vi "ni579x Synchronization Registers.vi"(0 "register instruction":T3, 5 "sync.resources":T1) -> (4 "read completion":T2, 14 "ready for input":bool)   [LabVIEW 2015, in "ni579x Synchronization v2 FPGA.lvlib"]
doc: "Set/get the configuration values for the Synchronization library by connecting it to the Register Bus.\n\n<B>Input Parameters</B>\n\n<B>register instruction</B> specifies a read or write register instruction. This parameter is usually obtained from the 'register instruction' parameter of the Process VI in the Register Bus FPGA library. The source of this parameter defines the instances of the Register Bus library to which the Synchronization library instance is wired, and is communicated from the host.\n\n<B>sync.resources</B> identifies the Synchronization instance. 'sync.resources' is obtained from the ni579x Create VI of this library.\n\n<B>Output Parameters</B>\n\n<B>read completion</B> indicates whether the register read operation has completed and returns the value for the register read.\n\n<B>ready for input</B> indicates whether the VI is ready to accept new input data in the next cycle. Use a Feedback Node to wire this parameter to the 'ready for output' terminal of an upstream node."
uses:
  <instrlib>/ni579x/Synchronization/v2/FPGA/ni579x Synchronization v2 FPGA.lvlib
  <instrlib>/_niInstr/Register Bus/v1/FPGA/Public/Register Instruction.ctl
  <instrlib>/_niInstr/Register Bus/v1/FPGA/Public/Read Completion.ctl
  <instrlib>/ni579x/Synchronization/v2/FPGA/Implementation/Resources.ctl
  <instrlib>/ni579x/Config/v2/Shared/Types/ni579x Register Bus Subsystem ID.ctl
  <instrlib>/_niInstr/Register Bus/v1/FPGA/niInstr Register Bus v1 FPGA.lvlib
  <instrlib>/ni579x/Config/v2/Shared/ni579x Config v2 Shared.lvlib
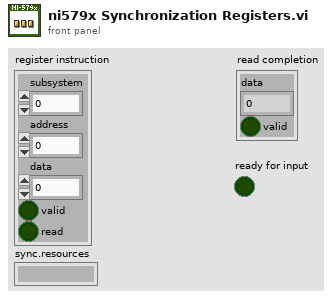
[diagram p1: front panel]
types:
  T1 = typedef "ni579x Synchronization v2 FPGA.lvlib/Resources.ctl" = cluster{"master":refnum<k21>, "meas.enable":refnum<k21>, "meas.ready":refnum<k21>, "meas.arm":refnum<k21>, "meas.valid":refnum<k21>, "meas.value":refnum<k21>, "meas.oversample clock":refnum<k21>, "meas.oversample factor":refnum<k21>, "cptr":refnum<k21>, "cptr.adjust":refnum<k21>, "cptr.period":refnum<k21>}
  T2 = typedef "niInstr Register Bus v1 FPGA.lvlib/Read Completion.ctl" = cluster{"data":u32, "valid":bool}
  T3 = typedef "niInstr Register Bus v1 FPGA.lvlib/Register Instruction.ctl" = cluster{"subsystem":u8, "address":u16, "data":u32, "valid":bool, "read":bool}
  T4 = typedef "ni579x Config v2 Shared.lvlib/ni579x Register Bus Subsystem ID.ctl" = u8
  T5 = typedef "ni579x Synchronization Register Addresses.ctl" = enum16{"Signature", "Current Version", "Oldest Compatible Version", "Scratch Register", "sync.master", "sync.meas.enable", "sync.meas.ready", "sync.meas.arm", "sync.meas.valid", "sync.meas.value", "sync.cptr.adjust", "sync.cptr.period", "sync.meas.oversample factor"}
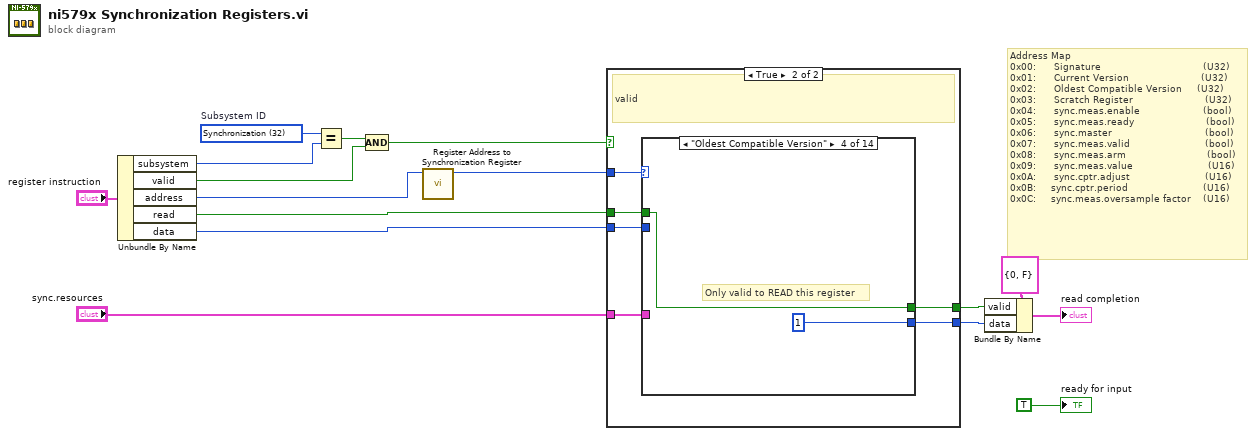
[diagram p0: block diagram]
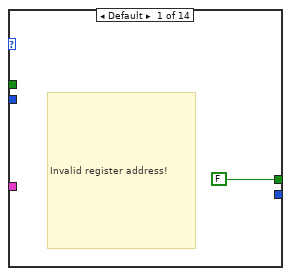
[diagram p3: hidden frame]
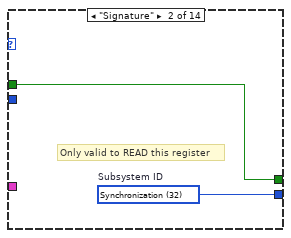
[diagram p4: hidden frame]
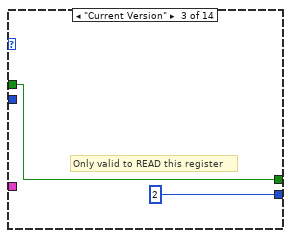
[diagram p5: hidden frame]
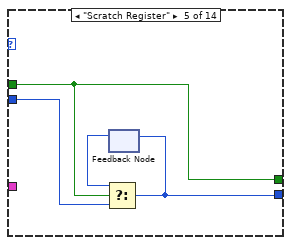
[diagram p6: hidden frame]
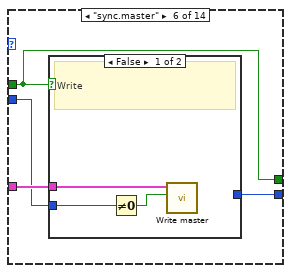
[diagram p7: hidden frame]
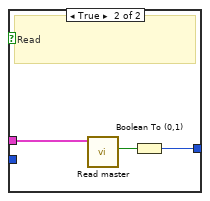
[diagram p8: hidden frame]
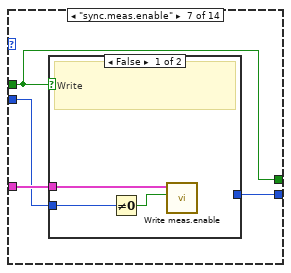
[diagram p9: hidden frame]
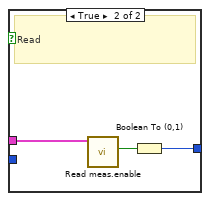
[diagram p10: hidden frame]
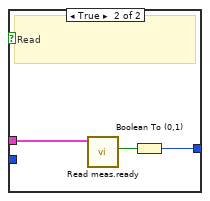
[diagram p12: hidden frame]
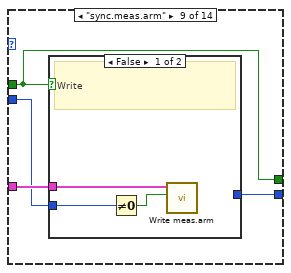
[diagram p13: hidden frame]
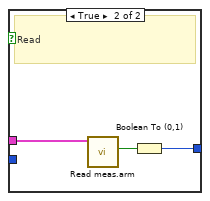
[diagram p14: hidden frame]
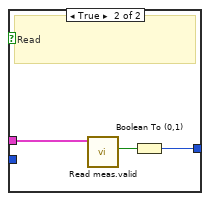
[diagram p16: hidden frame]
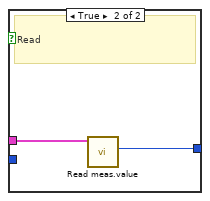
[diagram p18: hidden frame]
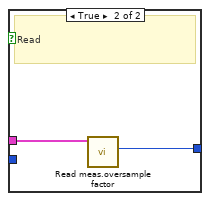
[diagram p20: hidden frame]
diagram:
  w12 = T4 32 items=["FAM Register Operation"=0, "User Command"=16, "Synchronization"=32]  # Subsystem ID
  # "Address Map\n0x00:      Signature                                  (U32)\n0x01:      Current Version                        (U32)\n0x02:      Oldest Compatible Version     (U32)\n0x03:      Scratch Register                        (U32)\n0x04:      sync.meas.enable                     (bool)\n0x05:      sync.meas.ready                        (bool)\n0x06:      sync.master                               (bool)\n0x07:      sync.meas.valid                         (bool)\n0x08:      sync.meas.arm                           (bool)\n0x09:      sync.meas.value                         (U16)\n0x0A:      sync.cptr.adjust                         (U16)\n0x0B:     sync.cptr.period                         (U16)\n0x0C:     sync.meas.oversample factor    (U16)"
  n1 = Unbundle By Name("register instruction") -> ("subsystem"=w4:u8, "valid"=w3:bool, "address"=w8:u16, "read"=w11:bool, "data"=w2:u32)
  n2 = Equal?(x=w12, y=w4) -> (x = y?=w13:bool)
  n3 = Compound Arithmetic op=AND(w13, w3) -> (w6:bool)
  n4 = call <instrlib>:"Register Address to Synchronization Register.vi"("address"=w8) -> ("register"=w7:T5)  [unwired: 10 in]
  n5 = case shown="True" w6 {
    selector: w6 -> [w17 _]
    tunnel: w11 -> [_ w23]
    tunnel: [_ w22] -> w10
    tunnel: w2 -> [_ w21]
    tunnel: w7 -> [_ w20]
    tunnel: "sync.resources" -> [_ w19]
    tunnel: [w17 w18] -> w1
    frame False {
      # "invalid"
    }
    frame True {
      # "valid"
      n6 = case shown="\"Oldest Compatible Version\"" w20 {
        tunnel: w23 -> [_ w25 w27 w29 w31 w35 w45 w55 w62 w72 w79 w85 w91 w100]
        tunnel: [_ w26 u32 2 ("data") u32 1 ("data") w33 w38 w48 w58 w65 w75 w82 w88 w94 w103] -> w22
        tunnel: w21 -> [_ _ _ _ w34 w36 w46 w56 w63 w73 w80 w86 w92 w101]
        tunnel: w19 -> [_ _ _ _ _ w37 w47 w57 w64 w74 w81 w87 w93 w102]
        tunnel: [FALSE w25 w27 w29 w31 w35 w45 w55 w62 w72 w79 w85 w91 w100] -> w18
        frame Default {
          # "Invalid register address!"
        }
        frame "Signature" {
          w26 = T4 32 items=["FAM Register Operation"=0, "User Command"=16, "Synchronization"=32]  # Subsystem ID
          # "Only valid to READ this register"
          # "Signature"
        }
        frame "Current Version" {
          # "Only valid to READ this register"
        }
        frame "Oldest Compatible Version" {
          # "Only valid to READ this register"
        }
        frame "Scratch Register" {
          n7 = feedback #1() -> (w32:u32)  [unwired: 1 in]
          n8 = Select(t=w32, s=w31, f=w34) -> (s? t:f=w33:u32)
          n9 = feedback-in #1(w33) -> ()
        }
        frame "sync.master" {
          n10 = case shown="False" w35 {
            tunnel: [_ w43] -> w38
            tunnel: w37 -> [w41 w42]
            tunnel: w36 -> [w40 _]
            frame False {
              # "Write"
              n11 = Not Equal To 0?(x=w40) -> (x != 0?=w39:bool)
              n12 = call <instrlib>:"Write master.vi"("master"=w39, "sync.resources"=w41) -> ()  [unwired: 9 in, 1 out]
            }
            frame True {
              # "Read"
              n13 = call <instrlib>:"Read master.vi"("sync.resources"=w42) -> ("master"=w44:bool)  [unwired: 9 in, 1 out]
              n14 = Boolean To (0,1)(Boolean=w44) -> (0, 1=w43:i16)
            }
          }
        }
        frame "sync.meas.enable" {
          n15 = case shown="False" w45 {
            tunnel: [_ w53] -> w48
            tunnel: w47 -> [w51 w52]
            tunnel: w46 -> [w50 _]
            frame False {
              # "Write"
              n16 = Not Equal To 0?(x=w50) -> (x != 0?=w49:bool)
              n17 = call <instrlib>:"Write meas.enable.vi"("meas.enable"=w49, "sync.resources"=w51) -> ()  [unwired: 9 in, 1 out]
            }
            frame True {
              # "Read"
              n18 = call <instrlib>:"Read meas.enable.vi"("sync.resources"=w52) -> ("meas.enable"=w54:bool)  [unwired: 9 in, 1 out]
              n19 = Boolean To (0,1)(Boolean=w54) -> (0, 1=w53:i16)
            }
          }
        }
        frame "sync.meas.ready" {
          n20 = case shown="False" w55 {
            tunnel: [_ w60] -> w58
            tunnel: w57 -> [_ w59]
            tunnel: w56 -> [_ _]
            frame False {
              # "Not allowed to write.\n\nThis register is written interally only."
              # "Write"
            }
            frame True {
              # "Read"
              n21 = call <instrlib>:"Read meas.ready.vi"("sync.resources"=w59) -> ("meas.ready"=w61:bool)  [unwired: 9 in, 1 out]
              n22 = Boolean To (0,1)(Boolean=w61) -> (0, 1=w60:i16)
            }
          }
        }
        frame "sync.meas.arm" {
          n23 = case shown="False" w62 {
            tunnel: [_ w70] -> w65
            tunnel: w64 -> [w68 w69]
            tunnel: w63 -> [w67 _]
            frame False {
              # "Write"
              n24 = Not Equal To 0?(x=w67) -> (x != 0?=w66:bool)
              n25 = call <instrlib>:"Write meas.arm.vi"("meas.arm"=w66, "sync.resources"=w68) -> ()  [unwired: 9 in, 1 out]
            }
            frame True {
              # "Read"
              n26 = call <instrlib>:"Read meas.arm.vi"("sync.resources"=w69) -> ("meas.arm"=w71:bool)  [unwired: 9 in, 1 out]
              n27 = Boolean To (0,1)(Boolean=w71) -> (0, 1=w70:i16)
            }
          }
        }
        frame "sync.meas.valid" {
          n28 = case shown="False" w72 {
            tunnel: [_ w77] -> w75
            tunnel: w74 -> [_ w76]
            tunnel: w73 -> [_ _]
            frame False {
              # "Not allowed to write.\n\nThis register is written interally only."
              # "Write"
            }
            frame True {
              # "Read"
              n29 = call <instrlib>:"Read meas.valid.vi"("sync.resources"=w76) -> ("meas.valid"=w78:bool)  [unwired: 9 in, 1 out]
              n30 = Boolean To (0,1)(Boolean=w78) -> (0, 1=w77:i16)
            }
          }
        }
        frame "sync.meas.value" {
          n31 = case shown="False" w79 {
            tunnel: [_ w83] -> w82
            tunnel: w81 -> [_ w84]
            tunnel: w80 -> [_ _]
            frame False {
              # "Not allowed to write.\n\nThis register is written interally only."
              # "Write"
            }
            frame True {
              # "Read"
              n32 = call <instrlib>:"Read meas.value.vi"("sync.resources"=w84) -> ("meas.value"=w83:u16)  [unwired: 9 in, 1 out]
            }
          }
        }
        frame "sync.meas.oversample factor" {
          n33 = case shown="False" w85 {
            tunnel: [_ w89] -> w88
            tunnel: w87 -> [_ w90]
            tunnel: w86 -> [_ _]
            frame False {
              # "Not allowed to write.\n\nThis register is written interally only."
              # "Write"
            }
            frame True {
              # "Read"
              n34 = call <instrlib>:"Read meas.oversample factor.vi"("sync.resources"=w90) -> ("meas.oversample factor"=w89:u16)  [unwired: 9 in, 1 out]
            }
          }
        }
        frame "sync.cptr.adjust" {
          n35 = case shown="False" w91 {
            tunnel: [_ w98] -> w94
            tunnel: w93 -> [w97 w99]
            tunnel: w92 -> [w96 _]
            frame False {
              # "Write"
              n36 = To Unsigned Word Integer(number=w96) -> (unsigned 16bit integer=w95:u16)
              n37 = call <instrlib>:"Write cptr.adjust.vi"("cptr.adjust"=w95, "sync.resources"=w97) -> ()  [unwired: 9 in, 1 out]
            }
            frame True {
              # "Read"
              n38 = call <instrlib>:"Read cptr.adjust.vi"("sync.resources"=w99) -> ("cptr.adjust"=w98:u16)  [unwired: 9 in, 1 out]
            }
          }
        }
        frame "sync.cptr.period" {
          n39 = case shown="False" w100 {
            tunnel: [_ w107] -> w103
            tunnel: w102 -> [w106 w108]
            tunnel: w101 -> [w105 _]
            frame False {
              # "Write"
              n40 = To Unsigned Word Integer(number=w105) -> (unsigned 16bit integer=w104:u16)
              n41 = call <instrlib>:"Write cptr.period.vi"("cptr.period"=w104, "sync.resources"=w106) -> ()  [unwired: 9 in, 1 out]
            }
            frame True {
              # "Read"
              n42 = call <instrlib>:"Read cptr.period.vi"("sync.resources"=w108) -> ("cptr.period"=w107:u16)  [unwired: 9 in, 1 out]
            }
          }
        }
      }
    }
  }
  n43 = Bundle By Name(cluster=T2 {"data"=0, "valid"=FALSE} ("read completion"), "valid"=w1, "data"=w10) -> (→"read completion":T2)
  "ready for input" <- TRUE ("ready for input")
